vi "发送数据记录到文档(子VI).vi"(7 "错误输入":errorcluster, 10 "数组":string[](array[string])) -> (0 "错误输出":errorcluster)   [LabVIEW 2016, in "数据传输系统.lvlib"]
uses:
  <vilib>/Utility/sysdir.llb/System Directory Type.ctl
panel:
  out "路径":path
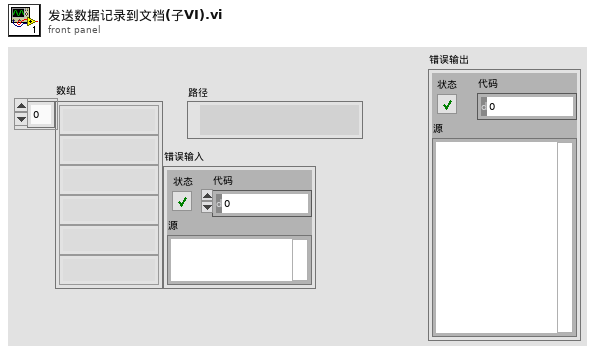
[diagram p1: front panel]
types:
  T1 = typedef "System Directory Type.ctl" = i32
  T2 = enum16{"open", "replace", "create", "open or create", "replace or create", "replace or create with confirmation"}
  T3 = typedef "LVDateTimeRec.ctl" = cluster{"秒数的小数部分":dbl, "秒":i32, "分":i32, "时":i32, "日":i32, "月":i32, "年":i32, "天数（周）":i32, "天数（年）":i32, "DST":i32}
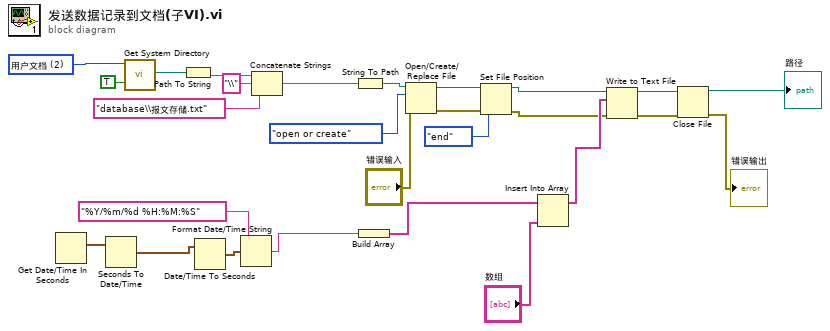
[diagram p0: block diagram]
diagram:
  w18 = T1 2 items=["用户目录"=0, "用户桌面"=1, "用户文档"=2, "用户应用程序数据"=3, "用户设置"=4, "用户临时目录"=5, "公共文档"=6, "公共应用程序数据"=7, "公共设置"=8, "公共缓存"=13, "系统核心库"=9, "系统安装库"=10, "应用程序文件"=11, "启动盘根目录"=12] ("system directory type")
  n1 = Get Date/Time In Seconds() -> (seconds since 1Jan1904=w5:timestamp)
  n2 = Seconds To Date/Time(time stamp (now)=w5) -> (date time rec=w2:T3)  [unwired: 1 in]
  n3 = call <vilib>:"Get System Directory.vi"("create directory if not found? (F)"=TRUE, "system directory type"=w18) -> ("system directory"=w16:path)  [unwired: 9 in]
  n4 = Path To String(path=w16) -> (string=w15:string)
  n5 = Date/Time To Seconds(2:w2) -> (0:w4:timestamp)  [unwired: 1 in]
  n6 = Format Date/Time String(time format string (%c)="%Y/%m/%d %H:%M:%S" ("时间格式字符串(%c)"), seconds (now)=w4) -> (date/time string=w1:string)  [unwired: 1 in]
  n7 = Concatenate Strings(w15, "\\" ("字符串"), "database\\报文存储.txt" ("字符串")) -> (w12:string)
  n8 = String To Path(string=w12) -> (path=w23:path)
  n9 = Build Array(w1) -> (w6:string[])
  n10 = Open/Create/Replace File(file path (use dialog)=w23, error in="错误输入", operation (0:open)=T2."open or create" ("操作(0:open)")) -> (refnum out=w11:refnum<file>, error out=w10:errorcluster)  [unwired: 3 in, 1 out]
  n11 = Set File Position(refnum=w11, from (0:start)=enum16{"start", "end", "current"}."end" ("自（0:起始）"), error in=w10) -> (refnum out=w9:refnum<file>, error out=w8:errorcluster)  [unwired: 1 in]
  n12 = Insert Into Array(array=w6, new element="数组") -> (w21:string[])  [unwired: 1 in]
  n13 = Write to Text File(file (use dialog)=w9, text=w21, error in=w8) -> (refnum out=w26:refnum<file>, error out=w27:errorcluster)  [unwired: 1 in, 1 out]
  n14 = Close File(refnum=w26, error in=w27) -> (path=→"路径":path, error out=→"错误输出":errorcluster)
